vi "Broadcast Response.vi"(8 "error in (no error)":errorcluster, 9 "Acquired Result.lvclass":refnum<class "Acquired Result.lvclass">, 10 "Topic":string, 11 "Measure Object in":refnum<class "Spectrum Recorder too.lvclass">) -> (0 "error out":errorcluster, 3 "Measure Object out":refnum<class "Spectrum Recorder too.lvclass">)   [LabVIEW 2018, in "Spectrum Recorder too.lvclass"]
uses:
  Spectrum Recorder too.lvclass
  C:/github/LabActor/Template Module/Template Module.lvclass
  NHMFL_Core/Libraries/Instruments/Results/Acquired Result/Acquired Result.lvclass
  NHMFL_Core/Libraries/Instruments/Results/Acquired Result/Acquired Result.lvclass/Acquired Result.ctl
  Template Module/Template Module.lvclass/Template Module.ctl
  NHMFL_Core/Libraries/Instruments/Results/Acquired Result/Write Group.vi
  Template Module/Read Logger.vi
  Template Module/Write Logger.vi
  Loggers/Logger/Logger.lvclass
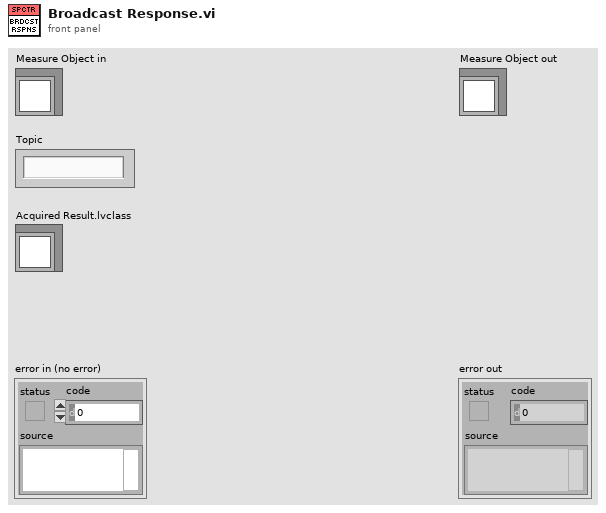
[diagram p1: front panel]
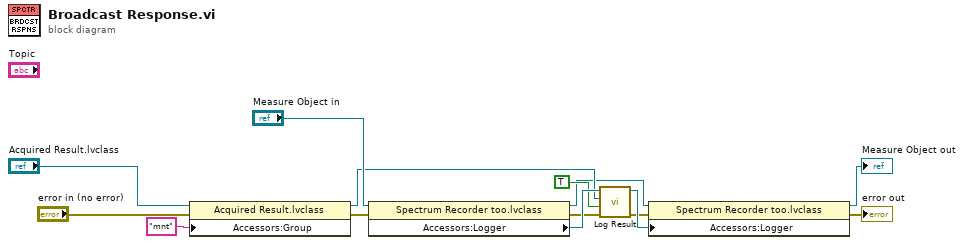
[diagram p0: block diagram]
diagram:
  n1 = property class="Acquired Result.lvclass"(reference="Acquired Result.lvclass", error in="error in (no error)", "Accessors:Group"="mnt" ("Group")) -> (reference out=w7:refnum<class "Acquired Result.lvclass">, error out=w9:errorcluster)
  n2 = property class="Spectrum Recorder too.lvclass"(reference="Measure Object in", error in=w9) -> (reference out=w2:refnum<class "Spectrum Recorder too.lvclass">, error out=w8:errorcluster, "Accessors:Logger"=w13:refnum<class "Logger.lvclass">)
  n3 = call-dynamic "Log Result.vi"("error in (no error)"=w8, "Timestamp data points"=TRUE, "Result"=w7, "Logger in"=w13) -> ("error out"=w4:errorcluster, "Logger out"=w5:refnum<class "Logger.lvclass">)  [unwired: 6 in]
  n4 = property class="Spectrum Recorder too.lvclass"(reference=w2, error in=w4, "Accessors:Logger"=w5) -> (reference out=→"Measure Object out":refnum<class "Spectrum Recorder too.lvclass">, error out=→"error out":errorcluster)
